vi "enable_by_name.vi"(8 "error in (no error)":errorcluster caption="错误输入（无错误）", 10 "name":string, 11 "MotorSystem 输入":refnum<class "MotorSystem.lvclass">) -> (0 "error out":errorcluster caption="错误输出", 3 "MotorSystem 输出":refnum<class "MotorSystem.lvclass">)   [LabVIEW 2016, in "MotionControl.lvlib" / "MotorSystem.lvclass"]
uses:
  <userlib>/MotionControl/MotorSystem/MotorSystem.lvclass
  <userlib>/MotionControl/MotorSystem/MotorSystem.lvclass/MotorSystem.ctl
  <userlib>/MotionControl/OneMotion/OneMotion.lvclass
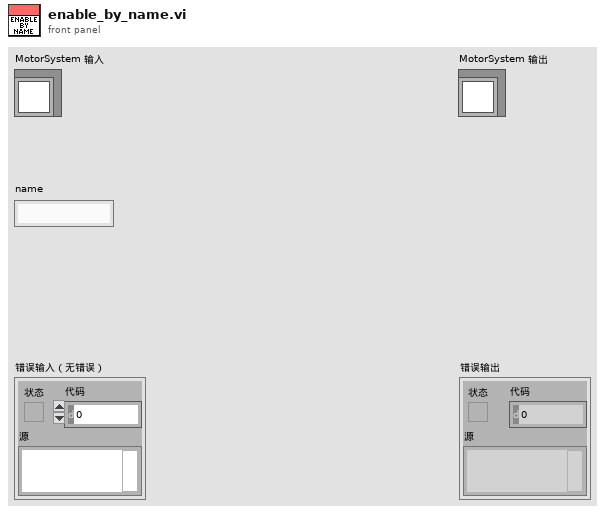
[diagram p1: front panel]
types:
  T1 = typedef "MotionControl.lvlib/MotorSystem.lvclass/MotionCluster.ctl" = cluster{"OneMotion.lvclass":refnum<class "OneMotion.lvclass">, "connected?":bool, "default enabled?":bool, "enabled?":bool}
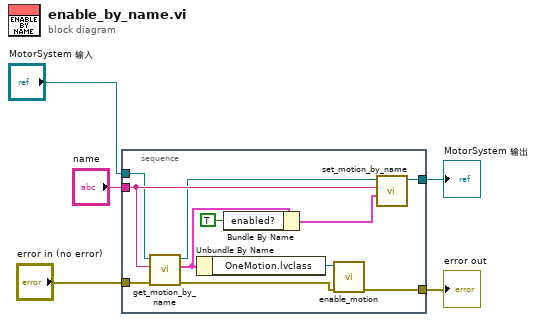
[diagram p0: block diagram]
diagram:
  n1 = stacked-sequence {
    tunnel: [w13] -> w5
    tunnel: [w6] -> w3
    tunnel: "MotorSystem 输入" -> [w7]
    tunnel: "error in (no error)" -> [w16]
    tunnel: "name" -> [w10]
    frame #0 {
      n2 = call <userlib>:"get_motion_by_name.vi"("error in (no error)"=w16, "name"=w10, "MotorSystem in"=w7) -> ("error out"=w14:errorcluster, "motion cluster"=w12:T1, "MotorSystem out"=w9:refnum<class "MotorSystem.lvclass">)  [unwired: 6 in]
      n3 = Unbundle By Name(w12) -> ("OneMotion.lvclass"=w15:refnum<class "OneMotion.lvclass">)
      n4 = Bundle By Name(cluster=w12, "enabled?"=TRUE) -> (w8:T1)
      n5 = call <userlib>:"enable_motion.vi"("error in (no error)"=w14, "OneMotion 输入"=w15) -> ("error out"=w13:errorcluster)  [unwired: 8 in, 1 out]
      n6 = call <userlib>:"set_motion_by_name.vi"("簇"=w8, "name"=w10, "MotorSystem输入"=w9) -> ("MotorSystem输出"=w6:refnum<class "MotorSystem.lvclass">)  [unwired: 7 in, 1 out]
    }
  }
  "error out" <- w5
  "MotorSystem 输出" <- w3
